vi "Transfer ID to Tree Items.vi"(8 "error in (no error)":errorcluster, 9 "Transfer ID":string, 10 "Indent":i32, 11 "Refnum in":T1) -> (0 "error out":errorcluster, 2 "Items":T2(array[cluster]), 3 "Refnum out":T1)   [LabVIEW 2017]
uses:
  DSF Configuration API/1.0.0/Public/Controls/DSF Config Data RefNum.ctl
  Tree Item Type.ctl
  DSF Configuration API/1.0.0/Public/Read Item/Read Transfer.vi
  DSF Configuration API/1.0.0/Public/Read Item/Read Settings.vi
  DSF Configuration API/1.0.0/DSF Configuration API.lvlib
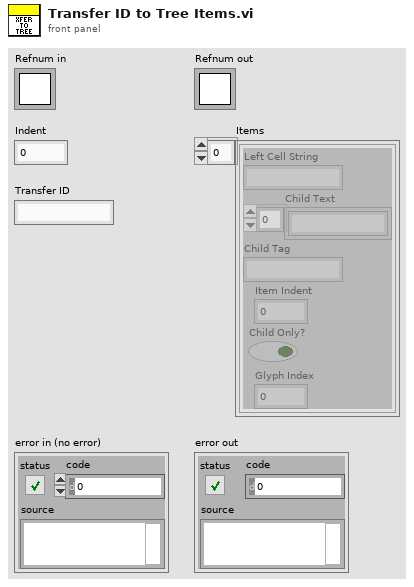
[diagram p1: front panel]
types:
  T1 = typedef "DSF Configuration API.lvlib/DSF Config Data RefNum.ctl" = refnum<k1>
  T2 = cluster{"Left Cell String":string, "Child Text":string[], "Child Tag":string, "Item Indent":i32, "Child Only?":bool, "Glyph Index":i32}[]
  T3 = typedef "Tree Item Type.ctl" = enum16{"Plugin", "Group", "Transfer", "Channel", "Setting"}
  T4 = typedef "DSF Configuration API.lvlib/DSF Transfer Info.ctl" = cluster{"byte order":i32, "channel ids":string[], "settings id":string}
  T5 = cluster{"Left Cell String":string, "Child Text":string[], "Child Tag":string, "Item Indent":i32, "Child Only?":bool, "Glyph Index":i32}
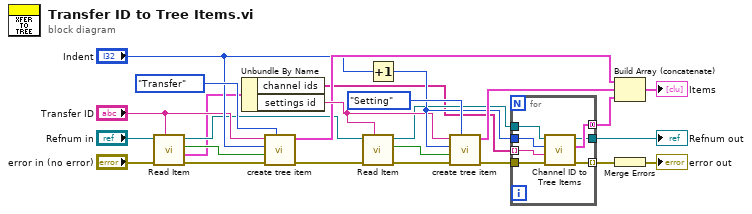
[diagram p0: block diagram]
diagram:
  n1 = call-poly "Read Item.vi"("name"="Transfer ID", "error in (no error)"="error in (no error)", "refnum"="Refnum in") -> ("error out"=w19:errorcluster, "value"=w1:T4, "found?"=w11:bool, "refnum out"=w4:T1)  [unwired: 5 in]
  n2 = Unbundle By Name(w1) -> ("channel ids"=w2:string[], "settings id"=w13:string)
  n3 = call "create tree item.vi"("Item Type"=Tree_Item_Type."Transfer", "error in"=w19, "found?"=w11, "Indent"="Indent", "Left Cell String"="Transfer ID") -> ("error out"=w20:errorcluster, "Item"=w12:T5)  [unwired: 5 in]
  n4 = call-poly "Read Item.vi"("name"=w13, "error in (no error)"=w20, "refnum"=w4) -> ("error out"=w21:errorcluster, "found?"=w15:bool, "refnum out"=w6:T1)  [unwired: 5 in, 1 out]
  n5 = Increment(x="Indent") -> (x+1=w14:i32)
  n6 = call "create tree item.vi"("Item Type"=Tree_Item_Type."Setting", "error in"=w21, "found?"=w15, "Indent"=w14, "Left Cell String"=w13) -> ("error out"=w22:errorcluster, "Item"=w16:T5)  [unwired: 5 in]
  n7 = for {
    tunnel: w2 -> [w30] mode=indexing
    tunnel: w6 -> [w32]
    tunnel: w22 -> [w31]
    tunnel: [w28] -> w7 mode=indexing
    tunnel: w14 -> [w29]
    tunnel: [w27] -> w17 mode=concatenating
    tunnel: [w26] -> w25
    n8 = call "Channel ID to Tree Items.vi"("error in (no error)"=w31, "Channel ID"=w30, "Indent"=w29, "Refnum in"=w32) -> ("error out"=w28:errorcluster, "Items"=w27:T2, "Refnum out"=w26:T1)  [unwired: 5 in]
  }
  "Refnum out" <- w25
  n9 = Build Array (concatenate)(w12, w16, w17) -> (→"Items":T2)
  n10 = Merge Errors(w7) -> (→"error out":errorcluster)
